vi "Add Point.vi"(8 "error in (no error)":errorcluster, 9 "X":dbl, 10 "Y":dbl, 11 "ExpFitter in":refnum<class "ExpFitter.lvclass">) -> (0 "error out":errorcluster, 3 "ExpFitter out":refnum<class "ExpFitter.lvclass">)   [LabVIEW 2019, in "ExpFitter.lvclass"]
uses:
  ExpFitter.lvclass
  ExpFitter.lvclass/ExpFitter.ctl
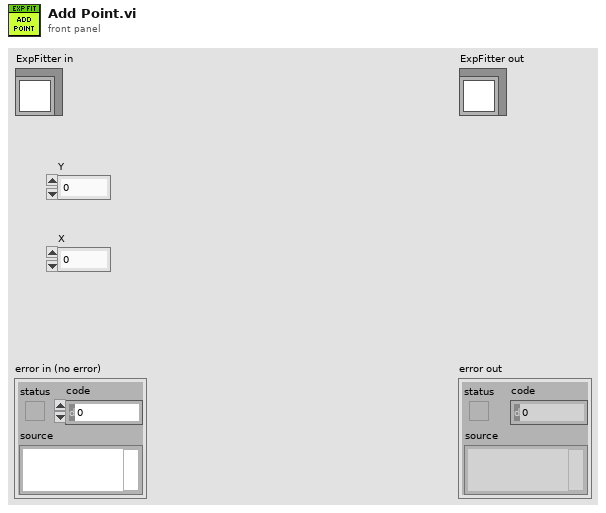
[diagram p1: front panel]
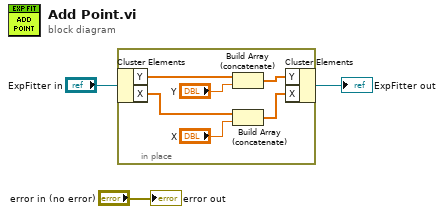
[diagram p0: block diagram]
diagram:
  n1 = in-place {
    n2 = in-place-cluster #1("ExpFitter in") -> ("Y"=w9:dbl[], "X"=w5:dbl[])
    n3 = Build Array (concatenate)(w9, "Y") -> (w8:dbl[])
    n4 = Build Array (concatenate)(w5, "X") -> (w4:dbl[])
    n5 = in-place-cluster #1("Y"=w8, "X"=w4) -> (→"ExpFitter out":refnum<class "ExpFitter.lvclass">)
  }
  "error out" <- "error in (no error)"
